vi "Data Validation.vi"(6 "Final Functional Test Station?":bool, 7 "Input Data Descriptor":T1, 8 "error in (no error)":errorcluster, 9 "Is HEX String?":bool, 10 "Input to Validate":string, 11 "Sequence Context In":refnum<k7>) -> (0 "error out":errorcluster, 2 "Message":string, 3 "String Valid?":bool)   [LabVIEW 2010]
uses:
  Data to Validate.ctl
  <vilib>/addons/TestStand/_TSUtility.llb/TestStand - Get Property Value (String).vi
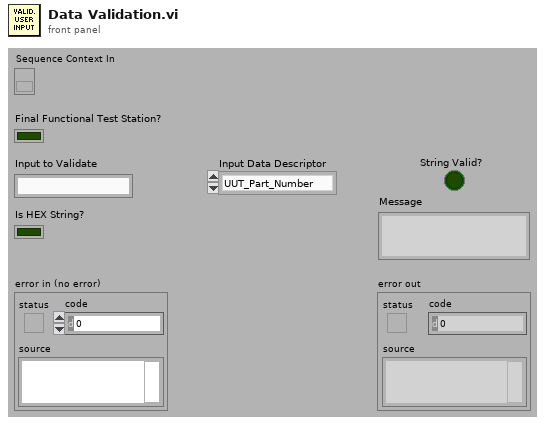
[diagram p1: front panel]
types:
  T1 = typedef "Data to Validate.ctl" = enum16{"UUT_Part_Number", "UUT_Serial_Number", "QiG_Serial_Number", "UUT_Model_Number", "UUT_Lot_Number", "Work_Order_Number", "UUT_MICS_ID"}
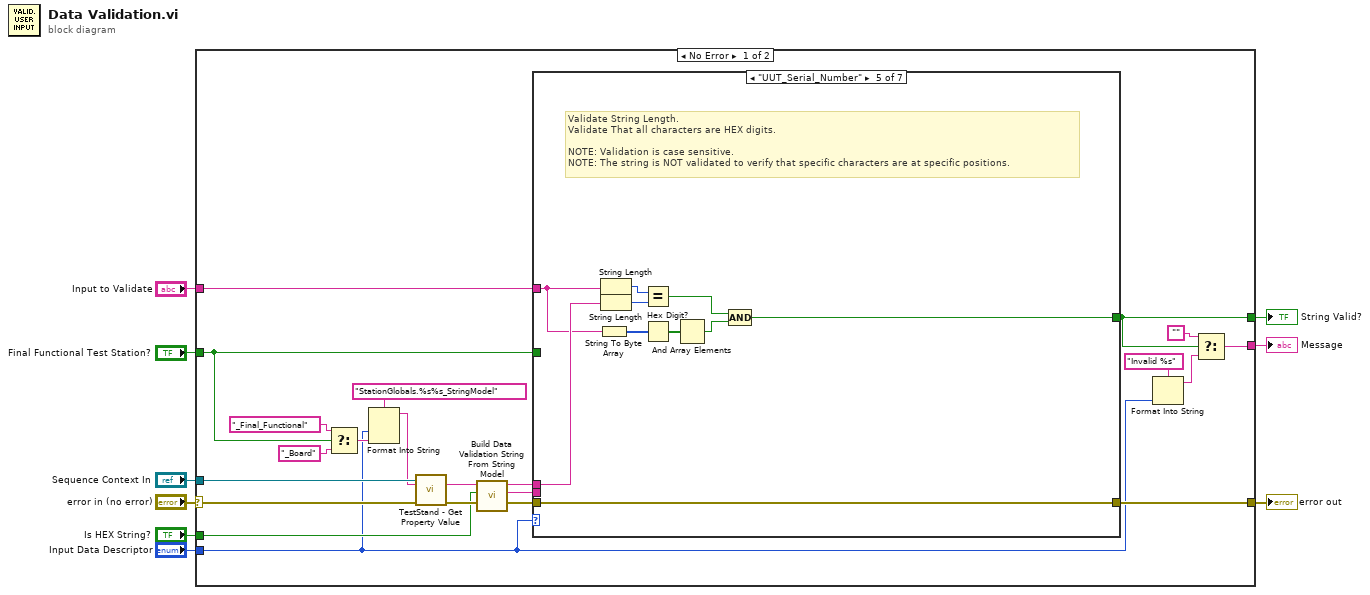
[diagram p0: block diagram]
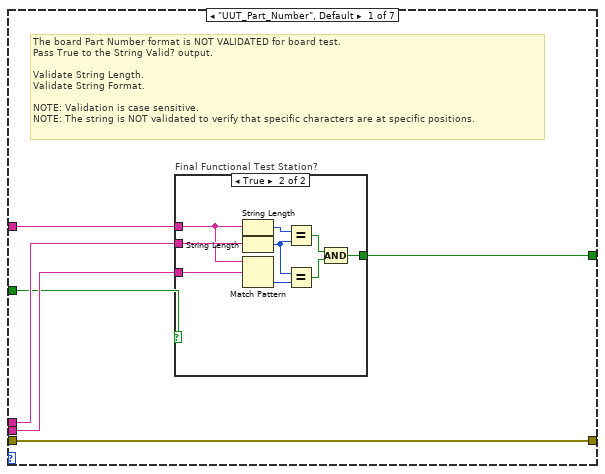
[diagram p2: hidden frame]
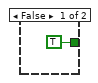
[diagram p3: hidden frame]
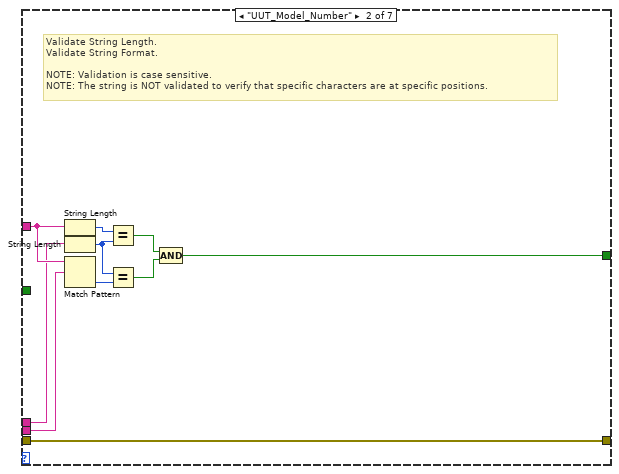
[diagram p4: hidden frame]
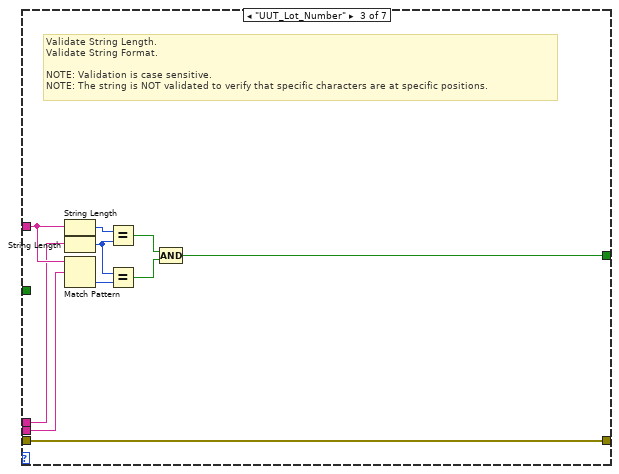
[diagram p5: hidden frame]
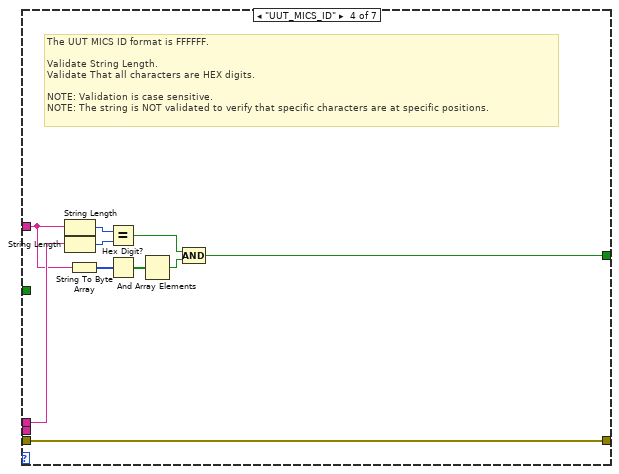
[diagram p6: hidden frame]
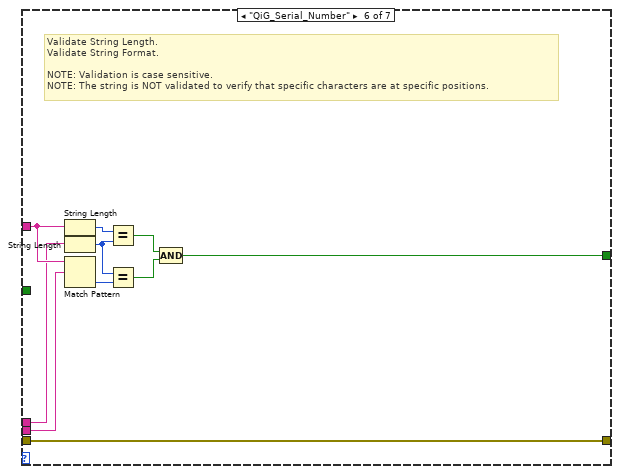
[diagram p7: hidden frame]
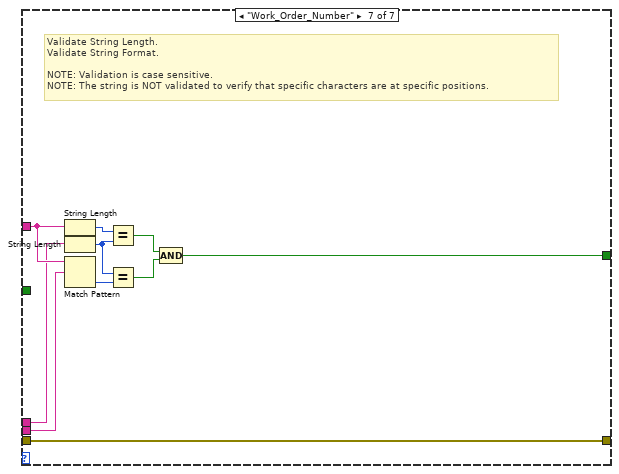
[diagram p8: hidden frame]
diagram:
  n1 = case shown="No Error" "error in (no error)" {
    selector: "error in (no error)" -> [w30 w107]
    tunnel: [w25 w107] -> w8
    tunnel: "Input Data Descriptor" -> [w11 _]
    tunnel: "Sequence Context In" -> [w28 _]
    tunnel: "Input to Validate" -> [w24 _]
    tunnel: [w18 _] -> w4
    tunnel: "Is HEX String?" -> [w20 _]
    tunnel: [w19 _] -> w2
    tunnel: "Final Functional Test Station?" -> [w10 _]
    frame No Error {
      n2 = Select(t="_Final_Functional", s=w10, f="_Board") -> (s? t:f=w12:string)
      n3 = Format Into String(format string="StationGlobals.%s%s_StringModel" ("initial string"), w11, w12) -> (resulting string=w27:string)  [unwired: 2 in, 1 out]
      n4 = call-poly <vilib>:"TestStand - Get Property Value.vi"("Sequence Context In"=w28, "Lookup String"=w27, "error in (no error)"=w30) -> ("Value"=w23:string, "error out"=w26:errorcluster)  [unwired: 10 in, 1 out]
      n5 = call "Build Data Validation String From String Model.vi"("String Model is HEX?"=w20, "String Model In"=w23) -> ("Regular Expression"=w21:string, "String Model Out"=w22:string)  [unwired: 8 in]
      n6 = case shown="\"UUT_Serial_Number\"" w11 {
        tunnel: w26 -> [w36 w56 w66 w76 w86 w96 w106]
        tunnel: [w36 w56 w66 w76 w86 w96 w106] -> w25
        tunnel: w22 -> [w34 w48 w58 w71 w79 w88 w98]
        tunnel: w24 -> [w32 w53 w63 w67 w78 w93 w103]
        tunnel: [w35 w49 w59 w72 w77 w89 w99] -> w18
        tunnel: w21 -> [w33 w47 w57 _ _ w87 w97]
        tunnel: w10 -> [w31 _ _ _ _ _ _]
        frame "UUT_Part_Number", Default {
          # "The board Part Number format is NOT VALIDATED for board test.\nPass True to the String Valid? output.\n\nValidate String Length.\nValidate String Format.\n\nNOTE: Validation is case sensitive.\nNOTE: The string is NOT validated to verify that specific characters are at specific positions."
          n7 = case "Final Functional Test Station?" shown="True" w31 {
            tunnel: [TRUE w41] -> w35
            tunnel: w34 -> [_ w40]
            tunnel: w33 -> [_ w39]
            tunnel: w32 -> [_ w38]
            frame False {
            }
            frame True {
              n8 = String Length(string=w38) -> (length=w46:i32)
              n9 = String Length(string=w40) -> (length=w43:i32)
              n10 = Match Pattern(string=w38, regular expression=w39) -> (offset past match=w44:i32)  [unwired: 1 in, 3 out]
              n11 = Equal?(x=w46, y=w43) -> (x = y?=w45:bool)
              n12 = Equal?(x=w43, y=w44) -> (x = y?=w42:bool)
              n13 = Compound Arithmetic op=AND(w45, w42) -> (w41:bool)
            }
          }
        }
        frame "UUT_Model_Number" {
          # "Validate String Length.\nValidate String Format.\n\nNOTE: Validation is case sensitive.\nNOTE: The string is NOT validated to verify that specific characters are at specific positions."
          n14 = String Length(string=w53) -> (length=w55:i32)
          n15 = String Length(string=w48) -> (length=w51:i32)
          n16 = Match Pattern(string=w53, regular expression=w47) -> (offset past match=w52:i32)  [unwired: 1 in, 3 out]
          n17 = Equal?(x=w55, y=w51) -> (x = y?=w54:bool)
          n18 = Equal?(x=w51, y=w52) -> (x = y?=w50:bool)
          n19 = Compound Arithmetic op=AND(w54, w50) -> (w49:bool)
        }
        frame "UUT_Lot_Number" {
          # "Validate String Length.\nValidate String Format.\n\nNOTE: Validation is case sensitive.\nNOTE: The string is NOT validated to verify that specific characters are at specific positions."
          n20 = String Length(string=w63) -> (length=w65:i32)
          n21 = String Length(string=w58) -> (length=w61:i32)
          n22 = Match Pattern(string=w63, regular expression=w57) -> (offset past match=w62:i32)  [unwired: 1 in, 3 out]
          n23 = Equal?(x=w65, y=w61) -> (x = y?=w64:bool)
          n24 = Equal?(x=w61, y=w62) -> (x = y?=w60:bool)
          n25 = Compound Arithmetic op=AND(w64, w60) -> (w59:bool)
        }
        frame "UUT_MICS_ID" {
          # "The UUT MICS ID format is FFFFFF.\n\nValidate String Length.\nValidate That all characters are HEX digits.\n\nNOTE: Validation is case sensitive.\nNOTE: The string is NOT validated to verify that specific characters are at specific positions."
          n26 = String Length(string=w67) -> (length=w75:i32)
          n27 = String Length(string=w71) -> (length=w73:i32)
          n28 = String To Byte Array(string=w67) -> (unsigned byte array=w70:u8[])
          n29 = Equal?(x=w75, y=w73) -> (x = y?=w74:bool)
          n30 = Hex Digit?(1:w70) -> (0:w69:bool[])
          n31 = And Array Elements(Boolean array=w69) -> (logical AND=w68:bool)
          n32 = Compound Arithmetic op=AND(w74, w68) -> (w72:bool)
        }
        frame "UUT_Serial_Number" {
          # "Validate String Length.\nValidate That all characters are HEX digits.\n\nNOTE: Validation is case sensitive.\nNOTE: The string is NOT validated to verify that specific characters are at specific positions."
          n33 = String To Byte Array(string=w78) -> (unsigned byte array=w82:u8[])
          n34 = String Length(string=w78) -> (length=w85:i32)
          n35 = String Length(string=w79) -> (length=w83:i32)
          n36 = Equal?(x=w85, y=w83) -> (x = y?=w84:bool)
          n37 = Hex Digit?(1:w82) -> (0:w81:bool[])
          n38 = And Array Elements(Boolean array=w81) -> (logical AND=w80:bool)
          n39 = Compound Arithmetic op=AND(w84, w80) -> (w77:bool)
        }
        frame "QiG_Serial_Number" {
          # "Validate String Length.\nValidate String Format.\n\nNOTE: Validation is case sensitive.\nNOTE: The string is NOT validated to verify that specific characters are at specific positions."
          n40 = String Length(string=w93) -> (length=w95:i32)
          n41 = String Length(string=w88) -> (length=w91:i32)
          n42 = Match Pattern(string=w93, regular expression=w87) -> (offset past match=w92:i32)  [unwired: 1 in, 3 out]
          n43 = Equal?(x=w95, y=w91) -> (x = y?=w94:bool)
          n44 = Equal?(x=w91, y=w92) -> (x = y?=w90:bool)
          n45 = Compound Arithmetic op=AND(w94, w90) -> (w89:bool)
        }
        frame "Work_Order_Number" {
          # "Validate String Length.\nValidate String Format.\n\nNOTE: Validation is case sensitive.\nNOTE: The string is NOT validated to verify that specific characters are at specific positions."
          n46 = String Length(string=w103) -> (length=w105:i32)
          n47 = String Length(string=w98) -> (length=w101:i32)
          n48 = Match Pattern(string=w103, regular expression=w97) -> (offset past match=w102:i32)  [unwired: 1 in, 3 out]
          n49 = Equal?(x=w105, y=w101) -> (x = y?=w104:bool)
          n50 = Equal?(x=w101, y=w102) -> (x = y?=w100:bool)
          n51 = Compound Arithmetic op=AND(w104, w100) -> (w99:bool)
        }
      }
      n52 = Format Into String(format string="Invalid %s" ("initial string"), w11) -> (resulting string=w15:string)  [unwired: 2 in, 1 out]
      n53 = Select(t="", s=w18, f=w15) -> (s? t:f=w19:string)
    }
    frame Error {
    }
  }
  "error out" <- w8
  "String Valid?" <- w4
  "Message" <- w2
